vi "SVT Max Frequency Within Tolerances [IEC].vi"(8 "error in (no error)":errorcluster, 9 "class":enum16{"Class 1", "Class 2"}(ring), 10 "weighting":u16(ring) items=["Linear", "A-weighting", "B-weighting", "C-weighting"], 11 "sampling frequency [Hz]":dbl=51200.0 format="%.2f") -> (0 "error out":errorcluster, 3 "max freq within tolerances [Hz]":dbl format="%.2f")   [LabVIEW 2017, in "SoundVib_ABCWeighting.lvlib"]
doc: "Returns the maximum frequency within tolerances according to the ANSI S1.4-2014/IEC 61672:2013 standard and <B>sampling frequency [Hz]</B>, <B>weighting</B>, and <B>class</B>."
uses:
  <vilib>/addons/Sound and Vibration/svt_Weighting/SoundVib_ABCWeighting.lvlib
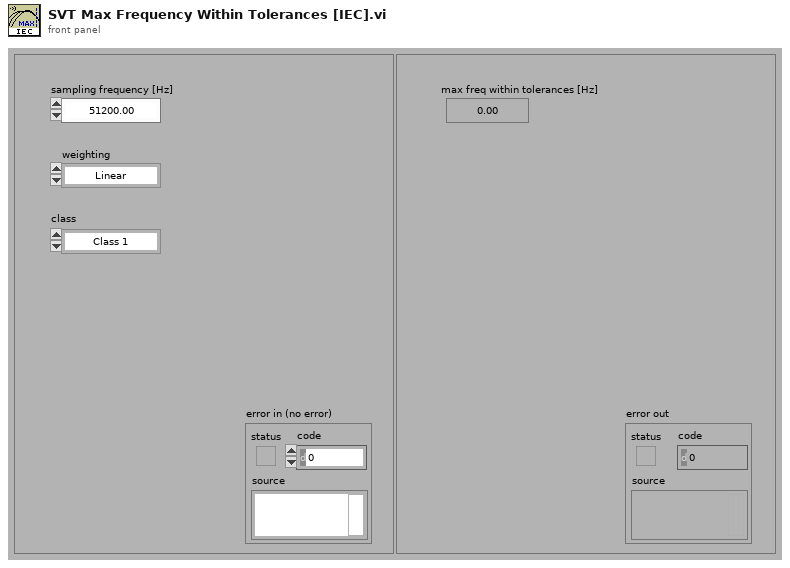
[diagram p1: front panel]
types:
  T1 = cluster{"filter structure":enum32{"IIR 2nd Order", "IIR 4th Order"}, "Reverse Coefficients":dbl[], "Forward Coefficients":dbl[]}
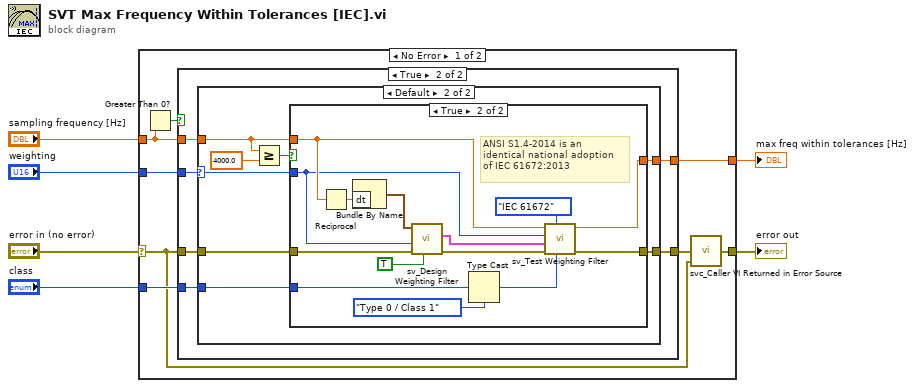
[diagram p0: block diagram]
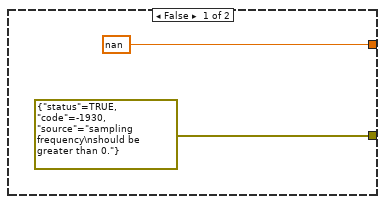
[diagram p2: hidden frame]
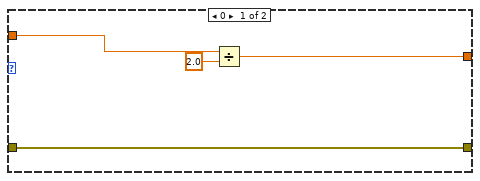
[diagram p3: hidden frame]
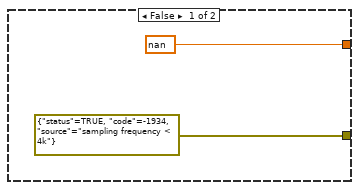
[diagram p4: hidden frame]
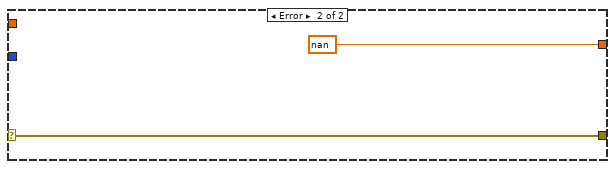
[diagram p5: hidden frame]
diagram:
  n1 = case shown="No Error" "error in (no error)" {
    selector: "error in (no error)" -> [w7 w52]
    tunnel: [w12 w52] -> w5
    tunnel: "weighting" -> [w14 _]
    tunnel: [w13 nan] -> w3
    tunnel: "sampling frequency [Hz]" -> [w8 _]
    tunnel: "class" -> [w11 _]
    frame No Error {
      n2 = Greater Than 0?(x=w8) -> (x > 0?=w10:bool)
      n3 = case shown="True" w10 {
        tunnel: w14 -> [_ w17]
        tunnel: [nan ("max freq within tolerances [Hz]") w20] -> w13
        tunnel: w8 -> [_ w18]
        tunnel: w11 -> [_ w19]
        tunnel: w7 -> [_ w22]
        tunnel: [errorcluster {"status"=TRUE, "code"=-1930, "source"="sampling frequency\nshould be greater than 0."} ("error in (no error)") w21] -> w9
        frame False {
        }
        frame True {
          n4 = case shown="Default" w17 {
            selector: w17 -> [_ w27]
            tunnel: w22 -> [w23 w34]
            tunnel: [w23 w33] -> w21
            tunnel: [w24 w32] -> w20
            tunnel: w19 -> [_ w31]
            tunnel: w18 -> [w25 w30]
            frame 0 {
              n5 = Divide(x=w25, y=2.0) -> (x/y=w24:dbl)
            }
            frame Default {
              n6 = Greater Or Equal?(x=w30, y=4000.0) -> (x >= y?=w28:bool)
              n7 = case shown="True" w28 {
                tunnel: w34 -> [_ w50]
                tunnel: [errorcluster {"status"=TRUE, "code"=-1934, "source"="sampling frequency < 4k"} ("error out") w46] -> w33
                tunnel: [nan ("max freq within tolerances [Hz]") w45] -> w32
                tunnel: w30 -> [_ w44]
                tunnel: w31 -> [_ w40]
                tunnel: w27 -> [_ w38]
                frame False {
                }
                frame True {
                  # "ANSI S1.4-2014 is an \nidentical national adoption \nof IEC 61672:2013"
                  n8 = Reciprocal(x=w44) -> (1/x=w49:dbl)
                  n9 = Bundle By Name("dt"=w49) -> (w48:waveform(dbl))  [unwired: 1 in]
                  n10 = call <vilib>:"sv_Design Weighting Filter.vi"("reset filter (F)"=TRUE, "error in (no error)"=w50, "weighting"=w38, "scaled signal"=w48) -> ("error out"=w47:errorcluster, "filter coefficients"=w39:T1)  [unwired: 5 in, 1 out]
                  n11 = Type Cast(type=enum16{"Type 0 / Class 1", "Type 1 / Class 2"}."Type 0 / Class 1" ("type or class"), x=w40) -> (*(type *) &x=w41:enum16{"Type 0 / Class 1", "Type 1 / Class 2"})
                  n12 = call <vilib>:"sv_Test Weighting Filter.vi"("type or class"=w41, "standard"=enum16{"ANSI S1.4", "IEC 61672"}."IEC 61672", "error in (no error)"=w47, "filter coefficients"=w39, "weighting"=w38, "sampling frequency [Hz]"=w44) -> ("error out"=w46:errorcluster, "max freq within tolerances [Hz]"=w45:dbl)  [unwired: 4 in]
                }
              }
            }
          }
        }
      }
      n13 = call <vilib>:"svc_Caller VI Returned in Error Source.vi"("warning input to caller"=w7, "error in (no error)"=w9) -> ("error out"=w12:errorcluster)  [unwired: 3 in]
    }
    frame Error {
    }
  }
  "error out" <- w5
  "max freq within tolerances [Hz]" <- w3
